vi "Make DLL Param(Read Batch Profile Advance Req).vi"(1 "Read Batch Profile Advance Req":T3 {"Batch Pos" items=["CURRENT", "SPECIFY", "COMMITED", "NEWEST PROFILE"]}) -> (0 "pReq":T2 {"Batch Pos" items=["CURRENT", "SPECIFY", "COMMITED", "NEWEST PROFILE"]})   [LabVIEW 8.6, in "Keyence LJ-V7000.lvlib"]
uses:
  Keyence LJ-V7000.lvlib
  Public/constant/Batch Pos.ctl
  Public/Clusters/Read Batch Profile Advance Req.ctl
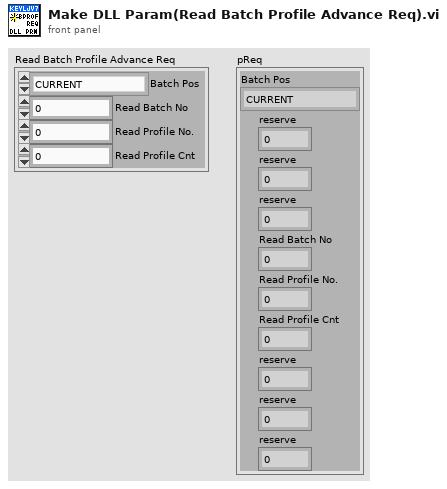
[diagram p1: front panel]
types:
  T1 = typedef "Keyence LJ-V7000.lvlib/Batch Pos.ctl" = u8
  T2 = cluster{"Batch Pos":T1, "reserve":u8, "reserve":u8, "reserve":u8, "Read Batch No":u32, "Read Profile No.":u32, "Read Profile Cnt":u8, "reserve":u8, "reserve":u8, "reserve":u8}
  T3 = typedef "Keyence LJ-V7000.lvlib/Read Batch Profile Advance Req.ctl" = cluster{"Batch Pos":T1, "Read Batch No":u32, "Read Profile No.":u32, "Read Profile Cnt":u8}
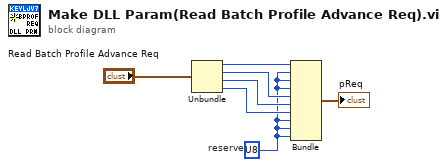
[diagram p0: block diagram]
diagram:
  w2 = u8 ?  # reserve
  n1 = Unbundle("Read Batch Profile Advance Req") -> ("Batch Pos"=w6:T1, "Read Batch No"=w5:u32, "Read Profile No."=w4:u32, "Read Profile Cnt"=w3:u8)
  n2 = Bundle("Batch Pos"=w6, "reserve"=w2, "reserve"=w2, "reserve"=w2, "Read Batch No"=w5, "Read Profile No."=w4, "Read Profile Cnt"=w3, "reserve"=w2, "reserve"=w2, "reserve"=w2) -> (→"pReq":T2)  [unwired: 1 in]
